vi "main.vi"() -> ()   [LabVIEW 2019]
panel:
  in  "Escala":i32
  in  "stop":bool
  out "rezise image":picture
  out "Original":picture
  in  "Path":path
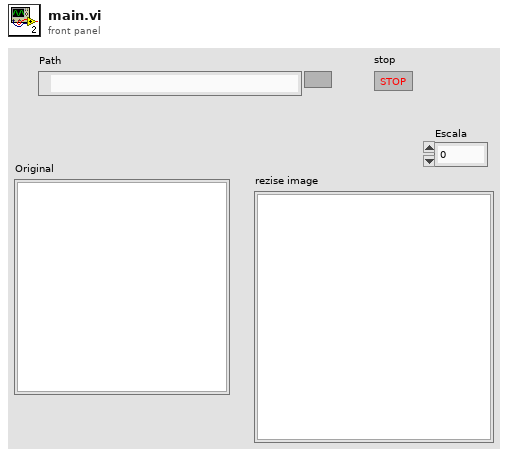
[diagram p1: front panel]
types:
  T1 = typedef "imagedata.ctl" = cluster{"image type":i32, "image depth":i32, "image":u8[], "mask":u8[], "colors":u32[], "Rectangle":cluster{"left":i16, "top":i16, "right":i16, "bottom":i16}}
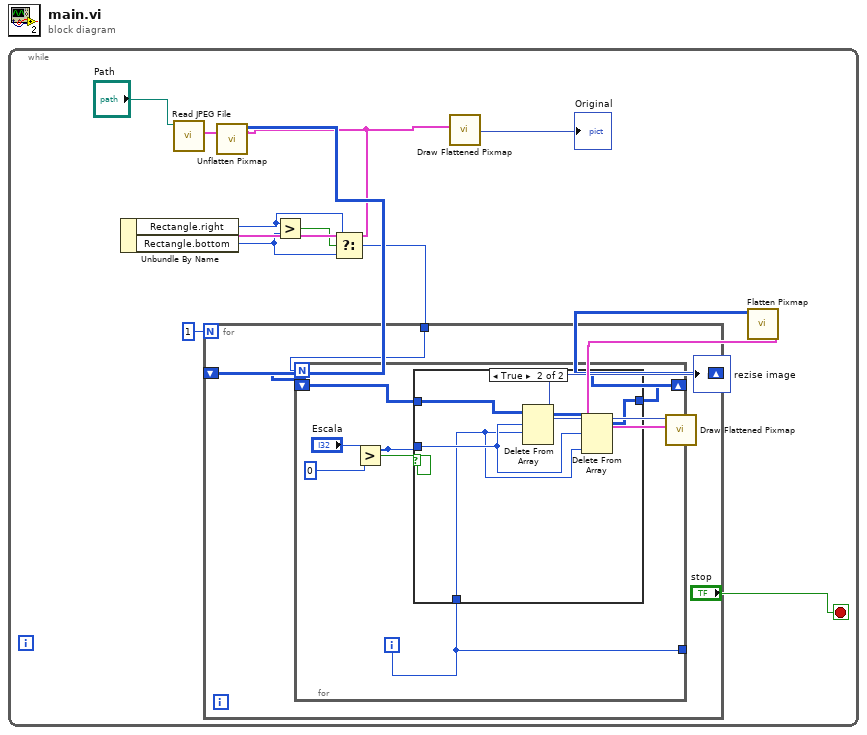
[diagram p0: block diagram]
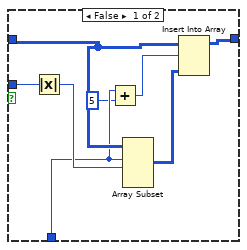
[diagram p2: hidden frame]
diagram:
  n1 = while {
    stop <- "stop" stop-if-true
    n2 = call <vilib>:"Read JPEG File.vi"("path to JPEG file"="Path") -> ("image data"=w6:T1)  [unwired: 8 in, 2 out]
    n3 = Unbundle By Name(w6) -> ("Rectangle.right"=w4:i16, "Rectangle.bottom"=w3:i16)
    n4 = call <vilib>:"Unflatten Pixmap.vi"("image data"=w6) -> ("24-bit pixmap"=w12:u32[][])  [unwired: 4 in, 6 out]
    n5 = Greater?(x=w4, y=w3) -> (0:w5:bool)
    n6 = Select(t=w4, s=w5, f=w3) -> (s? t:f=w2:i16)
    n7 = for {
      N: 1 -> [_]
      shift-right: [w15] -> w9
      shift-left: w12 -> [w16]
      tunnel: w2 -> [w14]
      n8 = for {
        N: w14 -> [_]
        tunnel: [w21] -> _
        shift-right: [w20] -> w15
        shift-left: w16 -> [w22]
        i -> [w21]
        n9 = Greater?(x="Escala", y=0) -> (0:w19:bool)
        n10 = case shown="True" w19 {
          tunnel: w22 -> [w27 w35]
          tunnel: w21 -> [w25 w31]
          tunnel: [w29 w33] -> w20
          tunnel: "Escala" -> [w30 w32]
          frame False {
            n11 = Absolute Value(x=w30) -> (abs(x)=w28:i32)
            n12 = Add(x=w25, y=5) -> (x+y=w24:i32)
            n13 = Array Subset(array=w27, index (row)=w25, length (row)=w28) -> (w26:u32[][])  [unwired: 2 in]
            n14 = Insert Into Array(array=w27, index (row)=w24, new element=w26) -> (w29:u32[][])  [unwired: 1 in]
          }
          frame True {
            n15 = Delete From Array(array=w35, length=w32, index (row)=w31) -> (array with subset deleted=w34:u32[][])  [unwired: 1 in, 1 out]
            n16 = Delete From Array(array=w34, length=w32, index (col)=w31) -> (array with subset deleted=w33:u32[][])  [unwired: 1 in, 1 out]
          }
        }
      }
    }
    n17 = call <vilib>:"Draw Flattened Pixmap.vi"("image data"=w6) -> ("new picture"=→"Original":picture)  [unwired: 8 in]
    n18 = call <vilib>:"Flatten Pixmap.vi"("24-bit pixmap"=w9) -> ("image data"=w11:T1)  [unwired: 10 in]
    n19 = call <vilib>:"Draw Flattened Pixmap.vi"("image data"=w11) -> ("new picture"=→"rezise image":picture)  [unwired: 8 in]
  }
